vi "WPI_CameraDiscoverAxisCameraIPs.vi"(8 "error in":errorcluster) -> (0 "error out":errorcluster, 3 "IP Addresses":string[](array[string]))   [LabVIEW 2017]
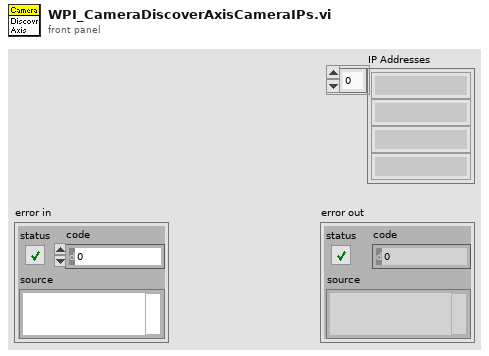
[diagram p1: front panel]
types:
  T1 = typedef "mdnsResolveInstance.ctl" = cluster{"name":string, "macAddress":string, "hostname":string, "ipAddress":string, "productId":string, "serialNumber":string, "systemStatus":string, "ifIndex":u32}
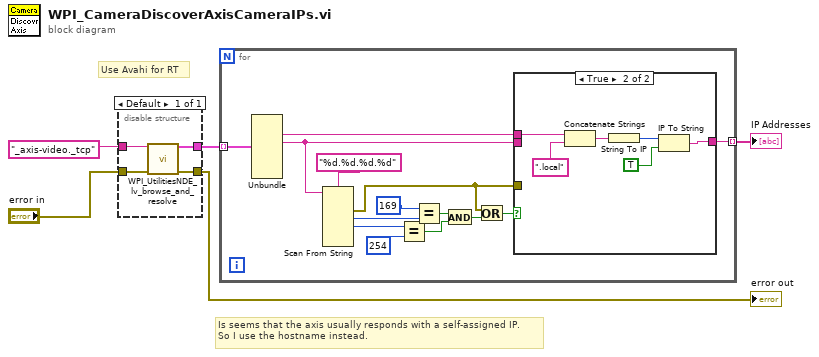
[diagram p0: block diagram]
diagram:
  # "Use Avahi for RT"
  # "Is seems that the axis usually responds with a self-assigned IP.\nSo I use the hostname instead."
  n1 = disable-structure shown="Default" {
    disable-tunnel: "_axis-video._tcp" ("serviceTypeName") -> [w9]
    disable-tunnel: [w8] -> w4
    disable-tunnel: [w7] -> w1
    disable-tunnel: "error in" -> [w6]
    frame Enabled {
      n2 = call <vilib>:"WPI_UtilitiesNDE_lv_browse_and_resolve.vi"("serviceTypeName"=w9, "error in"=w6) -> ("instances"=w8:T1[], "error out"=w7:errorcluster)  [unwired: 12 in]
    }
  }
  "error out" <- w1
  n3 = for {
    tunnel: w4 -> [w23] mode=indexing
    tunnel: [w13] -> w3 mode=indexing
    n4 = Unbundle(w23) -> ("hostname"=w15:string, "ipAddress"=w14:string)  [unwired: 6 out]
    n5 = Scan From String(format string="%d.%d.%d.%d" ("serviceTypeName"), input string=w14) -> (error out=w11:errorcluster, output 1=w21:i32, output 2=w18:i32)  [unwired: 8 in, 2 out]
    n6 = Equal?(x=w18, y=254 ("x")) -> (x = y?=w16:bool)
    n7 = Equal?(x=169, y=w21) -> (x = y?=w17:bool)
    n8 = And(x=w17, y=w16) -> (x .and. y?=w12:bool)
    n9 = Or(x=w11, y=w12) -> (x .or. y?=w10:bool)
    n10 = case shown="True" w10 {
      tunnel: w15 -> [_ w28]
      tunnel: w14 -> [w24 _]
      tunnel: [w24 w25] -> w13
      tunnel: w11 -> [_ _]
      frame False {
      }
      frame True {
        n11 = Concatenate Strings(w28, ".local" ("serviceTypeName")) -> (w30:string)
        n12 = String To IP(1:w30) -> (0:w27:u32)
        n13 = IP To String(1:TRUE ("dot notation? (F)"), 2:w27) -> (0:w25:string)
      }
    }
  }
  "IP Addresses" <- w3
